vi "Configure Peak Current Limits.vi"(0 "VISA resource name":refnum<visa-resource-name>, 5 "Current Peak Low Limit (0 A)":dbl min=0.0 max=220.8 format="%.3f", 7 "Current Peak High Limit (0 A)":dbl min=0.0 max=220.8 format="%.3f", 11 "error in (no error)":errorcluster) -> (4 "VISA resource name out":refnum<visa-resource-name>, 15 "error out":errorcluster)   [LabVIEW 2016, in "APT 300XAC Series.lvlib"]
doc: "Configures the current peak limits in the active step of the power source instrument.\n\n<B>Range</B> : 0.000~220.80 A\n\nVoltage Range = Low\n310XAC=0.0-36.8\n320XAC=0.0-73.6\n340XAC=0.0-147.2\n360XAC=0.0-220.8\n\nVoltage Range = High\n310XAC=0.0-18.4\n320XAC=0.0-36.8\n340XAC=0.0-73.6\n360XAC=0.0-110.4\n\n\n\nThe current peak Limit setting configures a peak current threshold level (High and Low Level). A test failure will occur when the high limit is reached or the low limit is not reached."
uses:
  APT 300XAC Series.lvlib
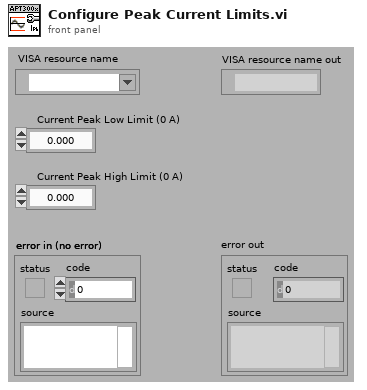
[diagram p1: front panel]
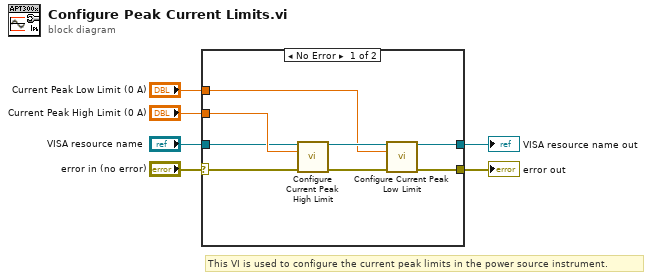
[diagram p0: block diagram]
diagram:
  # "This VI is used to configure the current peak limits in the power source instrument."
  n1 = case shown="No Error" "error in (no error)" {
    selector: "error in (no error)" -> [w7 w16]
    tunnel: [w13 w16] -> w6
    tunnel: [w12 w15] -> w5
    tunnel: "VISA resource name" -> [w8 w15]
    tunnel: "Current Peak High Limit (0 A)" -> [w10 _]
    tunnel: "Current Peak Low Limit (0 A)" -> [w9 _]
    frame No Error {
      n2 = call "Configure Current Peak High Limit.vi"("VISA resource name"=w8, "Current Peak High Limit (0 A)"=w10, "error in (no error)"=w7) -> ("VISA resource name out"=w11:refnum<visa-resource-name>, "error out"=w14:errorcluster)  [unwired: 11 in]
      n3 = call "Configure Current Peak Low Limit.vi"("VISA resource name"=w11, "Current Peak Low Limit (0 A)"=w9, "Error In"=w14) -> ("VISA resource name out"=w12:refnum<visa-resource-name>, "error out"=w13:errorcluster)  [unwired: 11 in]
    }
    frame Error {
    }
  }
  "error out" <- w6
  "VISA resource name out" <- w5
